vi "Config From Tree.vi"(8 "error in":errorcluster, 11 "XML in":string) -> (0 "error out":errorcluster, 1 "TargetIndex":i32, 2 "ProjectPath":path, 3 "XML out":string, 5 "Mode":T1)   [LabVIEW 2020]
uses:
  <vilib>/addons/analyzer/_analyzerctrls.llb/VIAnCtl AnalyzeMode.ctl
  <vilib>/addons/analyzer/_vianuishared.llb/VIAnUI CFG File Info Global.vi
  <vilib>/addons/analyzer/XML Parsing/NI_VIAn_XML Parsing.lvlib
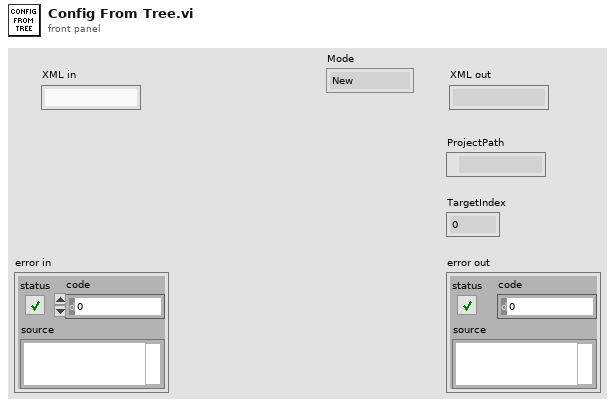
[diagram p1: front panel]
types:
  T1 = typedef "VIAnCtl AnalyzeMode.ctl" = enum16{"New", "Load", "AnalyzeThis", "AnalyzeProj"}
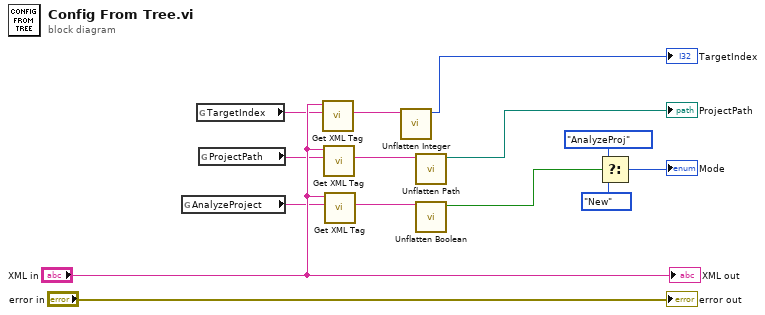
[diagram p0: block diagram]
diagram:
  n1 = global read "VIAnUI CFG File Info Global.vi" "AnalyzeProject"() -> (w7:string)
  n2 = global read "VIAnUI CFG File Info Global.vi" "TargetIndex"() -> (w9:string)
  n3 = global read "VIAnUI CFG File Info Global.vi" "ProjectPath"() -> (w8:string)
  n4 = call <vilib>:"Get XML Tag.vi"("Tag name"=w9, "XML String in"="XML in") -> ("Tag value"=w2:string)  [unwired: 5 in, 4 out]
  n5 = call <vilib>:"Get XML Tag.vi"("Tag name"=w8, "XML String in"="XML in") -> ("Tag value"=w4:string)  [unwired: 5 in, 4 out]
  n6 = call <vilib>:"Get XML Tag.vi"("Tag name"=w7, "XML String in"="XML in") -> ("Tag value"=w6:string)  [unwired: 5 in, 4 out]
  n7 = call <vilib>:"Unflatten Integer.vi"("Tag value"=w2) -> ("Numeric"=→"TargetIndex":i32)  [unwired: 10 in]
  n8 = call <vilib>:"Unflatten Path.vi"("Tag value"=w4) -> ("Path"=→"ProjectPath":path)  [unwired: 10 in]
  n9 = call <vilib>:"Unflatten Boolean.vi"("Tag value"=w6) -> ("Boolean"=w5:bool)  [unwired: 10 in]
  n10 = Select(t=VIAnCtl_AnalyzeMode."AnalyzeProj" ("Mode"), s=w5, f=VIAnCtl_AnalyzeMode."New" ("Mode")) -> (s? t:f=→"Mode":T1)
  "error out" <- "error in"
  "XML out" <- "XML in"
